vi "Gasflaschen Aenderung.vi"(7 "init":bool, 8 "Fehler (Eingang, kein Fehler)":errorcluster, 10 "TestKonfig alt":T1 {"TestKonfig Interferent"."Gasflasche MFC3" items=["----"=10000, "IAG NH3 3000"=0, "IAG NH3 200"=1, "IAG NH3 2000"=2, "IAG MG"=3, "IAG O2"=4]; "TestKonfig Interferent"."Gasflasche MFC2" items=["----"=10000, "IAG NH3 3000"=0, "IAG NH3 200"=1, "IAG NH3 2000"=2, "IAG MG"=3, "IAG O2"=4]; "TestKonfig Interferent"."Eingangs Konzentration MFC1" min=0.0; "TestKonfig Interferent"."Ausgangs Konzentration MFC1" min=0.0; "TestKonfig Interferent"."MFC2" items=["MFC 2", "MFC 3", "MFC 4", "MFC 5"]; "TestKonfig Interferent"."MFC3" items=["MFC 2", "MFC 3", "MFC 4", "MFC 5"]; "TestKonfig Interferent"."Ausgangs Konzentration MFC3" min=0.0; "TestKonfig Interferent"."Eingangs Konzentration MFC3" min=0.0; "TestKonfig Interferent"."Ausgangs Konzentration MFC2" min=0.0; "TestKonfig Interferent"."Eingangs Konzentration MFC2" min=0.0; "TestKonfig H2O"."HovaCAL Temperature" format="%.2f"; "TestKonfig H2O"."HovaCAL Flow Input Cluster"."HovaCAL Flow Input Cluster" format="%.2f"; "TestKonfig H2O"."Eingangs Konzentration:" min=0.0; "TestKonfig H2O"."zusätzliche Zeitdauer Erster Punkt" min=30 step=1 format="%#_5g"; "TestKonfig H2O"."Zeitdauer Stufen" format="%#_5g"; "TestKonfig H2O"."Max Fehler" format="%#_5g"; "TestKonfig H2O"."Anzahl Stufen" format="%#_5g"; "TestKonfig H2O"."Modus" items=["Messen", "CG zu Entnahmestelle"]}, 11 "TestKonfig (Eingang)":T1 {"TestKonfig Interferent"."Gasflasche MFC3" items=["----"=10000, "IAG NH3 3000"=0, "IAG NH3 200"=1, "IAG NH3 2000"=2, "IAG MG"=3, "IAG O2"=4]; "TestKonfig Interferent"."Gasflasche MFC2" items=["----"=10000, "IAG NH3 3000"=0, "IAG NH3 200"=1, "IAG NH3 2000"=2, "IAG MG"=3, "IAG O2"=4]; "TestKonfig Interferent"."Eingangs Konzentration MFC1" min=0.0; "TestKonfig Interferent"."Ausgangs Konzentration MFC1" min=0.0; "TestKonfig Interferent"."MFC2" items=["MFC 2", "MFC 3", "MFC 4", "MFC 5"]; "TestKonfig Interferent"."MFC3" items=["MFC 2", "MFC 3", "MFC 4", "MFC 5"]; "TestKonfig Interferent"."Ausgangs Konzentration MFC3" min=0.0; "TestKonfig Interferent"."Eingangs Konzentration MFC3" min=0.0; "TestKonfig Interferent"."Ausgangs Konzentration MFC2" min=0.0; "TestKonfig Interferent"."Eingangs Konzentration MFC2" min=0.0; "TestKonfig H2O"."HovaCAL Temperature" format="%.2f"; "TestKonfig H2O"."HovaCAL Flow Input Cluster"."HovaCAL Flow Input Cluster" format="%.2f"; "TestKonfig H2O"."Eingangs Konzentration:" min=0.0; "TestKonfig H2O"."zusätzliche Zeitdauer Erster Punkt" min=30 step=1 format="%#_5g"; "TestKonfig H2O"."Zeitdauer Stufen" format="%#_5g"; "TestKonfig H2O"."Max Fehler" format="%#_5g"; "TestKonfig H2O"."Anzahl Stufen" format="%#_5g"; "TestKonfig H2O"."Modus" items=["Messen", "CG zu Entnahmestelle"]}) -> (0 "Fehler (Ausgang)":errorcluster, 2 "TestKonfig alt out":T1 {"TestKonfig Interferent"."Gasflasche MFC3" items=["----"=10000, "IAG NH3 3000"=0, "IAG NH3 200"=1, "IAG NH3 2000"=2, "IAG MG"=3, "IAG O2"=4]; "TestKonfig Interferent"."Gasflasche MFC2" items=["----"=10000, "IAG NH3 3000"=0, "IAG NH3 200"=1, "IAG NH3 2000"=2, "IAG MG"=3, "IAG O2"=4]; "TestKonfig Interferent"."Eingangs Konzentration MFC1" min=0.0; "TestKonfig Interferent"."Ausgangs Konzentration MFC1" min=0.0; "TestKonfig Interferent"."MFC2" items=["MFC 2", "MFC 3", "MFC 4", "MFC 5"]; "TestKonfig Interferent"."MFC3" items=["MFC 2", "MFC 3", "MFC 4", "MFC 5"]; "TestKonfig Interferent"."Ausgangs Konzentration MFC3" min=0.0; "TestKonfig Interferent"."Eingangs Konzentration MFC3" min=0.0; "TestKonfig Interferent"."Ausgangs Konzentration MFC2" min=0.0; "TestKonfig Interferent"."Eingangs Konzentration MFC2" min=0.0; "TestKonfig H2O"."HovaCAL Temperature" format="%.2f"; "TestKonfig H2O"."HovaCAL Flow Input Cluster"."HovaCAL Flow Input Cluster" format="%.2f"; "TestKonfig H2O"."Eingangs Konzentration:" min=0.0; "TestKonfig H2O"."zusätzliche Zeitdauer Erster Punkt" min=30 step=1 format="%#_5g"; "TestKonfig H2O"."Zeitdauer Stufen" format="%#_5g"; "TestKonfig H2O"."Max Fehler" format="%#_5g"; "TestKonfig H2O"."Anzahl Stufen" format="%#_5g"; "TestKonfig H2O"."Modus" items=["Messen", "CG zu Entnahmestelle"]}, 3 "TestKonfig (Ausgang)":T1 {"TestKonfig Interferent"."Gasflasche MFC3" items=["----"=10000, "IAG NH3 3000"=0, "IAG NH3 200"=1, "IAG NH3 2000"=2, "IAG MG"=3, "IAG O2"=4]; "TestKonfig Interferent"."Gasflasche MFC2" items=["----"=10000, "IAG NH3 3000"=0, "IAG NH3 200"=1, "IAG NH3 2000"=2, "IAG MG"=3, "IAG O2"=4]; "TestKonfig Interferent"."Eingangs Konzentration MFC1" min=0.0; "TestKonfig Interferent"."Ausgangs Konzentration MFC1" min=0.0; "TestKonfig Interferent"."MFC2" items=["MFC 2", "MFC 3", "MFC 4", "MFC 5"]; "TestKonfig Interferent"."MFC3" items=["MFC 2", "MFC 3", "MFC 4", "MFC 5"]; "TestKonfig Interferent"."Ausgangs Konzentration MFC3" min=0.0; "TestKonfig Interferent"."Eingangs Konzentration MFC3" min=0.0; "TestKonfig Interferent"."Ausgangs Konzentration MFC2" min=0.0; "TestKonfig Interferent"."Eingangs Konzentration MFC2" min=0.0; "TestKonfig H2O"."HovaCAL Temperature" format="%.2f"; "TestKonfig H2O"."HovaCAL Flow Input Cluster"."HovaCAL Flow Input Cluster" format="%.2f"; "TestKonfig H2O"."Eingangs Konzentration:" min=0.0; "TestKonfig H2O"."zusätzliche Zeitdauer Erster Punkt" min=30 step=1 format="%#_5g"; "TestKonfig H2O"."Zeitdauer Stufen" format="%#_5g"; "TestKonfig H2O"."Max Fehler" format="%#_5g"; "TestKonfig H2O"."Anzahl Stufen" format="%#_5g"; "TestKonfig H2O"."Modus" items=["Messen", "CG zu Entnahmestelle"]})   [LabVIEW 2020, in "EPA 1065.lvlib" / "HovaCAL Interference verificaton.lvlib"]
uses:
  HovaCAL Interference verificaton.lvlib
  TestKonfig.ctl
  TestKonfig H2O.ctl
  Modus.ctl
  Linearisierung V2/SpanEinstellungen/Einheit.ctl
  Linearisierung V2/Gasteiler/Stufen Tabelle.ctl
  Linearisierung V2/Gasteiler/HovaCAL_Interface/Controls/Flow Einstellung.ctl
  Linearisierung V2/Gasteiler/HovaCAL_Interface/Controls/Temp Sollwerte Anzeige.ctl
  TestKonfig Interferents.ctl
  MFCAuswahl.ctl
  Seiten/System Einstellungen V2/Gasflasche Auswahl.ctl
  Linearisierung V2/SpanEinstellungen/SpanEinstellungen.lvlib
  Linearisierung V2/Gasteiler/Gasteiler.lvlib
  Seiten/System Einstellungen V2/System Einstellungen V2.lvlib
  Linearisierung V2/Gasteiler/HovaCAL_Interface/Controls/Controls.lvlib
panel:
  # "sec"
  # "%"
  # "sec"
  # "sec"
  # "%"
  # "sec"
  # "sec"
  # "%"
  # "sec"
  # "sec"
  # "%"
  # "sec"
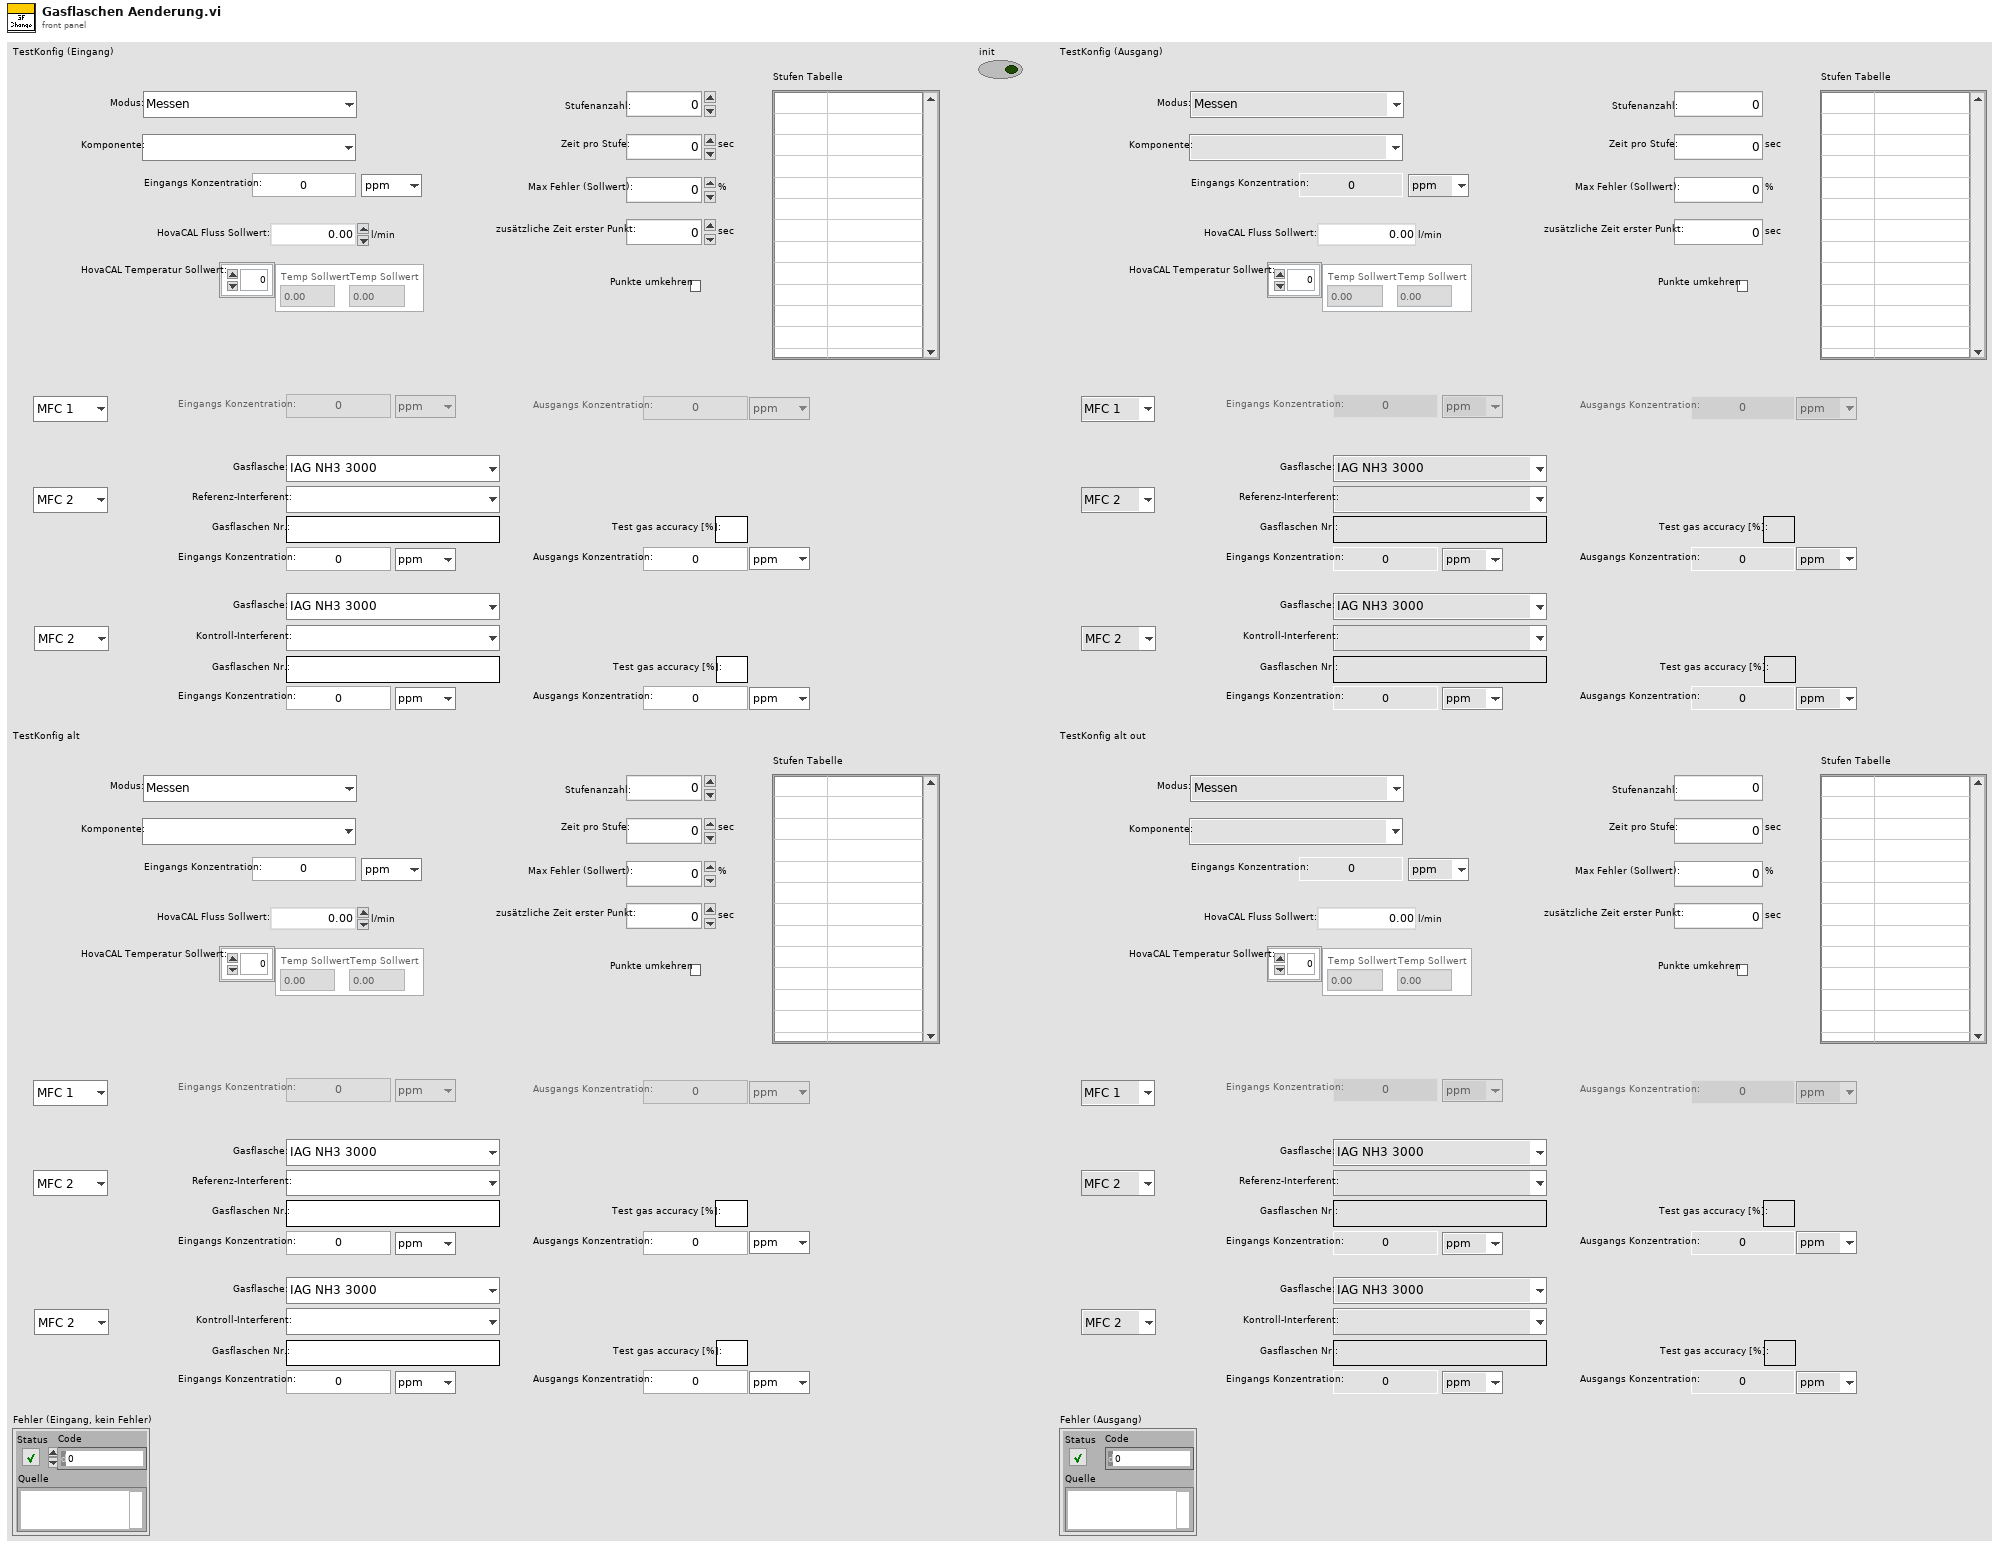
[diagram p1: front panel]
types:
  T1 = typedef "EPA 1065.lvlib/HovaCAL Interference verificaton.lvlib/TestKonfig.ctl" = cluster{"TestKonfig H2O":T2, "TestKonfig Interferent":T8}
  T2 = typedef "EPA 1065.lvlib/HovaCAL Interference verificaton.lvlib/TestKonfig H2O.ctl" = cluster{"Modus":T3, "Komponente:":u16, "Eingangs Konzentration:":dbl, "Einheit":T4, "Anzahl Stufen":sgl, "Zeitdauer Stufen":sgl, "Max Fehler":sgl, "zusätzliche Zeitdauer Erster Punkt":sgl, "Punkte umkehren":bool, "Stufen Tabelle":T5, "HovaCAL Flow Input Cluster":T6, "HovaCAL Temperature":T7}
  T3 = typedef "EPA 1065.lvlib/HovaCAL Interference verificaton.lvlib/Modus.ctl" = u16
  T4 = typedef "Linearisierung v2.lvlib/SpanEinstellungen.lvlib/Einheit.ctl" = enum16{"ppm", "%"}
  T5 = typedef "Linearisierung v2.lvlib/Gasteiler.lvlib/Stufen Tabelle.ctl" = string[][]
  T6 = typedef "Linearisierung v2.lvlib/Gasteiler.lvlib/HovaCAL_Interface.lvlib/Controls.lvlib/Flow Einstellung.ctl" = cluster{"HovaCAL Flow Input Cluster":dbl}
  T7 = typedef "Linearisierung v2.lvlib/Gasteiler.lvlib/HovaCAL_Interface.lvlib/Controls.lvlib/Temp Sollwerte Anzeige.ctl" = dbl[]
  T8 = typedef "EPA 1065.lvlib/HovaCAL Interference verificaton.lvlib/TestKonfig Interferents.ctl" = cluster{"MFC1":enum16{"MFC 1"}, "Eingangs Konzentration MFC1":dbl, "Einheit MFC1 Eingang":T4, "Ausgangs Konzentration MFC1":dbl, "Einheit MFC1 Ausgang":T4, "MFC2":T9, "Referenz-Interferent:":u16, "Gasflaschen Nr MFC2":string, "Accuracy MFC2":string, "Eingangs Konzentration MFC2":dbl, "Einheit MFC2 Eingang":T4, "Ausgangs Konzentration MFC2":dbl, "Einheit MFC2 Ausgang":T4, "MFC3":T9, "Kontroll-Interferent:":u16, "Gasflaschen Nr MFC3":string, "Accuracy MFC3":string, "Eingangs Konzentration MFC3":dbl, "Einheit MFC3 Eingang":T4, "Ausgangs Konzentration MFC3":dbl, "Einheit MFC3 Ausgang":T4, "Gasflasche MFC2":T10, "Gasflasche MFC3":T10}
  T9 = typedef "EPA 1065.lvlib/HovaCAL Interference verificaton.lvlib/MFCAuswahl.ctl" = u16
  T10 = typedef "System Einstellungen V2.lvlib/Gasflasche Auswahl.ctl" = u16
  T11 = typedef "EPA 1065.lvlib/HovaCAL Interference verificaton.lvlib/Konfig changes.ctl" = cluster{"Komp changes":bool, "MFC2 GF changed":bool, "MFC3 GF changed":bool, "MFC2 RefInterf changed":bool, "MFC3 KontrInterf changed":bool, "MFC2 GF ----":bool, "MFC3 GF ----":bool, "MFC2 Konzentration changed":bool, "MFC3 Konzentration changed":bool, "Einheiten changed":bool}
  T12 = cluster{"MFC2 Eingang":bool, "MFC2 Ausgang":bool, "MFC3 Eingang":bool, "MFC3 Ausgang":bool}
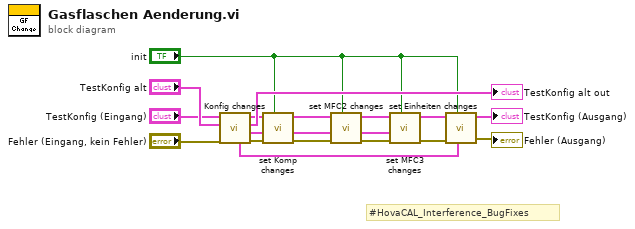
[diagram p0: block diagram]
diagram:
  # "#HovaCAL_Interference_BugFixes"
  n1 = call "Konfig changes.vi"("Fehler (Eingang, kein Fehler)"="Fehler (Eingang, kein Fehler)", "TestKonfig alt"="TestKonfig alt", "TestKonfig (Eingang)"="TestKonfig (Eingang)") -> ("Fehler (Ausgang)"=w13:errorcluster, "Changes"=w15:T11, "TestKonfig alt out"=→"TestKonfig alt out":T1, "TestKonfig (Ausgang)"=w16:T1, "Einheiten Changes-Cluster"=w1:T12)  [unwired: 4 in]
  n2 = call "set Komp changes.vi"("init"="init", "Fehler (Eingang, kein Fehler)"=w13, "Changes"=w15, "TestKonfig (Eingang) (Eingang)"=w16) -> ("Fehler (Ausgang)"=w14:errorcluster, "Changes  out"=w12:T11, "TestKonfig (Ausgang)"=w11:T1)  [unwired: 4 in, 1 out]
  n3 = call "set MFC2 changes.vi"("init"="init", "Fehler (Eingang, kein Fehler)"=w14, "Changes"=w12, "TestKonfig (Eingang)"=w11) -> ("Fehler (Ausgang)"=w8:errorcluster, "Changes  out"=w9:T11, "TestKonfig (Ausgang)"=w10:T1)  [unwired: 4 in, 1 out]
  n4 = call "set MFC3 changes.vi"("init"="init", "Fehler (Eingang, kein Fehler)"=w8, "Changes"=w9, "TestKonfig (Eingang)"=w10) -> ("Fehler (Ausgang)"=w4:errorcluster, "TestKonfig (Ausgang)"=w6:T1)  [unwired: 4 in, 2 out]
  n5 = call "set Einheiten changes.vi"("Einheiten Changes-Cluster"=w1, "init"="init", "Fehler (Eingang, kein Fehler)"=w4, "TestKonfig (Eingang)"=w6) -> ("Fehler (Ausgang)"=→"Fehler (Ausgang)":errorcluster, "TestKonfig (Ausgang)"=→"TestKonfig (Ausgang)":T1)  [unwired: 6 in]
